vi "Compile.vi"(8 "Error In":errorcluster, 11 "Compiler In":refnum<class "Compiler.lvclass">) -> (0 "Error Out":errorcluster, 3 "Compiler Out":refnum<class "Compiler.lvclass">)   [LabVIEW 2018, in "Toolkit.lvlib" / "Compiler.lvclass"]
uses:
  Compiler.lvclass
  Toolkit.lvlib
  Support/Render to String.vi
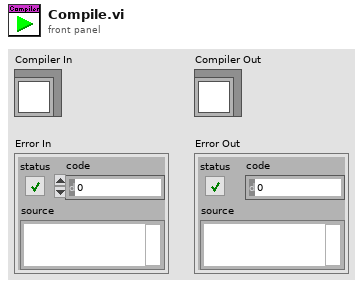
[diagram p1: front panel]
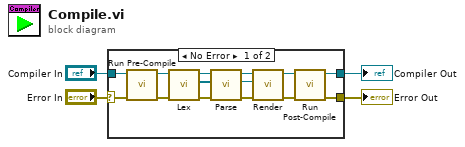
[diagram p0: block diagram]
diagram:
  n1 = case shown="No Error" "Error In" {
    selector: "Error In" -> [w13 w19]
    tunnel: "Compiler In" -> [w14 w20]
    tunnel: [w12 w20] -> w2
    tunnel: [w11 w19] -> w1
    frame No Error {
      n2 = call-dynamic "Run Pre-Compile.vi"("Error In"=w13, "Compiler In"=w14) -> ("Error Out"=w17:errorcluster, "Compiler Out"=w18:refnum<class "Compiler.lvclass">)  [unwired: 8 in]
      n3 = call-dynamic "Lex.vi"("Error In"=w17, "Compiler In"=w18) -> ("Error Out"=w8:errorcluster, "Tokens"=w7:refnum<class "Token.lvclass">[], "Compiler Out"=w10:refnum<class "Compiler.lvclass">)  [unwired: 7 in]
      n4 = call-dynamic "Parse.vi"("Error In"=w8, "Tokens"=w7, "Compiler In"=w10) -> ("Error Out"=w5:errorcluster, "Abstract Syntax Tree"=w6:refnum<class "Root.lvclass">, "Compiler Out"=w9:refnum<class "Compiler.lvclass">)  [unwired: 6 in]
      n5 = call-poly "Render.vi"("Error In"=w5, "Abstract Syntax Tree"=w6, "Context In"=w9) -> ("Error Out"=w15:errorcluster, "Context Out"=w16:refnum<class "Compiler.lvclass">)  [unwired: 6 in, 1 out]
      n6 = call-dynamic "Run Post-Compile.vi"("Error In"=w15, "Compiler In"=w16) -> ("Error Out"=w11:errorcluster, "Compiler Out"=w12:refnum<class "Compiler.lvclass">)  [unwired: 8 in]
    }
    frame Error {
    }
  }
  "Compiler Out" <- w2
  "Error Out" <- w1
